vi "Add Value Table to Channel.vi"(8 "error in (no error)":errorcluster, 10 "Value Table":string, 11 "Channel Ref":u64) -> (0 "error out":errorcluster, 3 "Channel Ref out":u64)   [LabVIEW 2025, in "Protection and Counter Addon System Explorer.lvlib"]
uses:
  Protection and Counter Addon System Explorer.lvlib
  <vilib>/NI/NI VeriStand Advanced SysDef API/SysDef API/Advanced System Definition.lvlib
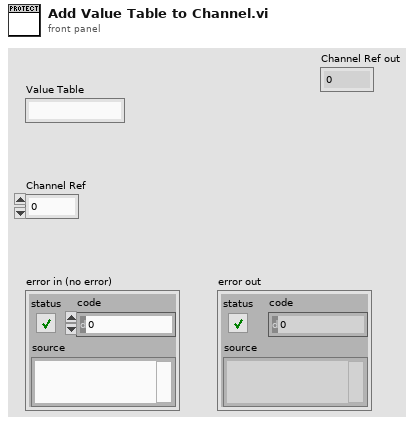
[diagram p1: front panel]
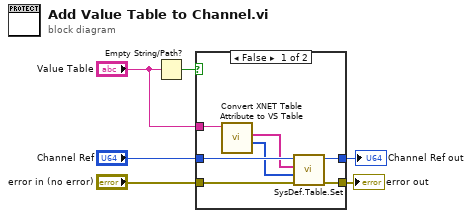
[diagram p0: block diagram]
diagram:
  n1 = Empty String/Path?(string/path="Value Table") -> (empty?=w2:bool)
  n2 = case shown="False" w2 {
    tunnel: "Channel Ref" -> [w13 w15]
    tunnel: [w12 w14] -> w4
    tunnel: [w11 w15] -> w1
    tunnel: "error in (no error)" -> [w10 w14]
    tunnel: "Value Table" -> [w9 _]
    frame False {
      n3 = call "Convert XNET Table Attribute to VS Table.vi"("attribute text"=w9) -> ("Value"=w7:i64[], "Names"=w8:string[])  [unwired: 9 in]
      n4 = call <vilib>:"SysDef.Table.Set.vi"("error in (no error)"=w10, "Values"=w7, "Names"=w8, "nodeID"=w13) -> ("error out"=w12:errorcluster, "nodeID out"=w11:u64)  [unwired: 6 in]
    }
    frame True {
    }
  }
  "error out" <- w4
  "Channel Ref out" <- w1
